vi "Streaming Xcvr (FPGA MODIFIED).vi"() -> ()   [LabVIEW 2015]
doc: "Acquires data from the Rx ports and streams the data to the host while receiving data from the host and generating the resulting waveform at the Tx ports of the NI USRP-294x/295x device. Use this VI as a template for the Simple NI-USRP Streaming sample project."
uses:
  <instrlib>/_niInstr/DSP/v1/Shared/Public/IQ Impairments.ctl
  SubVIs/Stream Control State.ctl
  Host/SubVIs/Start Trigger.ctl
  <instrlib>/_niInstr/DSP/v1/Shared/Public/IQ Gain.ctl
  <instrlib>/_niInstr/Register Bus/v1/FPGA/Public/Read Cmd Data.ctl
  SubVIs/DDC Parameters.ctl
  SubVIs/DUC Parameters.ctl
  <vilib>/Platform/TimedLoop/XDataNode/timing_clust.ctl
  <vilib>/Platform/TimedLoop/XDataNode/nitl_modes.ctl
  <vilib>/Platform/TimedLoop/XDataNode/wakeup.ctl
  <vilib>/rvi/Emulation/niFpgaGetClockAttributes.vi
  <vilib>/rvi/Emulation/niFpgaSctlEmulationGetInTimedLoop.vi
  <vilib>/rvi/Emulation/niFpgaEmulationReportErrorSimple.vi
  <vilib>/rvi/Emulation/niFpgaCriticalErrorInLSC.vi
  <vilib>/rvi/Emulation/niFpgaProcessEmulError.vi
  <vilib>/rvi/eio/common/nirviEmuTemplateMethod_errors.vi
  <vilib>/Platform/TimedLoop/XDataNode/XDataNode.xnode
  <vilib>/eio/EIONode/EIONode.xnode
  <vilib>/Platform/TimedLoop/XDataNode/XDNodeRunTimeDep.lvlib
  <instrlib>/_niInstr/Register Bus/v1/FPGA/niInstr Register Bus v1 FPGA.lvlib
  <instrlib>/_niInstr/DSP/v1/Shared/niInstr DSP v1 Shared.lvlib
  <instrlib>/niUsrpRio/Config/v1/FPGA/niUsrpRio Config v1 FPGA.lvlib
  FPGA Timekeeper.lvlib
  Host/PPS_Global_Var.vi
panel:
  out "FPGA Timekeeper time (ns)":u64
  out "FPGA Timekeeper locked":bool
  out "offset from time reference":i32
  out "PPS":bool
  in  "absolute time offset(ns)":u64
  in  "RF 1/Tx/Enable":bool
  in  "RF 1/Rx/Enable":bool
  in  "RF 0/Tx/Enable":bool
  in  "RF 0/Rx/Enable":bool
  out "tx.parameters":T5={"tx.trigger select"=enum."Software", "tx.trigger enable"=FALSE, "tx.trigger sync enable"=FALSE, "tx 0.stream enable"=FALSE, "tx 1.stream enable"=FALSE, "tx.software trigger"=FALSE, "tx.reset"=FALSE, "tx.abort"=FALSE, "tx.samples to generate"=0, "duc parameters"=[{"frequency shift"=0.0, "impairments"={"inline gain I"=0.0, "inline gain Q"=0.0, "cross gain I"=0.0, "cross gain Q"=0.0, "pre-gain offset I"=0.0, "pre-gain offset Q"=0.0, "post-gain offset I"=0.0, "post-gain offset Q"=0.0}, "phase"=0.0, "input sample rate"=0.0, "gain"={"gain I"=0.0, "gain Q"=0.0}, "delay"=0.0}, {"frequency shift"=0.0, "impairments"={"inline gain I"=0.0, "inline gain Q"=0.0, "cross gain I"=0.0, "cross gain Q"=0.0, "pre-gain offset I"=0.0, "pre-gain offset Q"=0.0, "post-gain offset I"=0.0, "post-gain offset Q"=0.0}, "phase"=0.0, "input sample rate"=0.0, "gain"={"gain I"=0.0, "gain Q"=0.0}, "delay"=0.0}]} {"duc parameters"."frequency shift" format="%#.48g"}
  out "tx.status":T7
  out "rx.status":T8
  out "rx.parameters":T10={"rx.trigger select"=enum."Software", "rx.trigger enable"=FALSE, "rx.trigger sync enable"=FALSE, "rx 0.stream enable"=FALSE, "rx 1.stream enable"=FALSE, "rx.software trigger"=FALSE, "rx.reset"=FALSE, "rx.abort"=FALSE, "rx.samples to acquire"=0, "ddc parameters"=[{"output sample rate"=0.0, "delay"=0.0, "frequency shift"=0.0, "impairments"={"inline gain I"=0.0, "inline gain Q"=0.0, "cross gain I"=0.0, "cross gain Q"=0.0, "pre-gain offset I"=0.0, "pre-gain offset Q"=0.0, "post-gain offset I"=0.0, "post-gain offset Q"=0.0}, "phase"=0.0}, {"output sample rate"=0.0, "delay"=0.0, "frequency shift"=0.0, "impairments"={"inline gain I"=0.0, "inline gain Q"=0.0, "cross gain I"=0.0, "cross gain Q"=0.0, "pre-gain offset I"=0.0, "pre-gain offset Q"=0.0, "post-gain offset I"=0.0, "post-gain offset Q"=0.0}, "phase"=0.0}]} {"ddc parameters"."frequency shift" format="%#.48g"}
  in  "TX DSP Settings Tab Control":T11(tab)=enum."TX Stream Settings"
  in  "tx.trigger enable":bool
  in  "tx.software trigger":bool
  in  "tx.trigger select":T1=enum."Immediate"
  in  "tx.trigger sync enable":bool
  in  "tx 0.stream enable":bool
  in  "tx 1.stream enable":bool
  in  "tx.reset":bool=TRUE
  in  "tx.abort":bool
  in  "tx.samples to generate":u32
  in  "tx.input sample rate":fxp<+,48,1>
  in  "tx.delay":fxp<+/-,18,0>
  out "tx.dsp reset done":bool
  out "tx.state":T6
  out "tx.number of fifo underflows":u32
  out "tx.samples processed":u32
  in  "tx 0.impairments":T3={"inline gain I"=0.9999923706054688, "inline gain Q"=0.9999923706054688, "cross gain I"=0.0, "cross gain Q"=0.0, "pre-gain offset I"=0.0, "pre-gain offset Q"=0.0, "post-gain offset I"=0.0, "post-gain offset Q"=0.0}
  in  "tx 0.frequency shift":fxp<+/-,48,0> format="%#.48g"
  in  "tx 0.phase":fxp<+/-,21,0>
  in  "tx 0.gain":T4={"gain I"=1.0, "gain Q"=1.0}
  out "tx 0.number of IQ data overflows":u64
  in  "tx 1.gain":T4={"gain I"=1.0, "gain Q"=1.0}
  in  "tx 1.phase":fxp<+/-,21,0>
  in  "tx 1.frequency shift":fxp<+/-,48,0> format="%#.48g"
  in  "tx 1.impairments":T3={"inline gain I"=0.9999923706054688, "inline gain Q"=0.9999923706054688, "cross gain I"=0.0, "cross gain Q"=0.0, "pre-gain offset I"=0.0, "pre-gain offset Q"=0.0, "post-gain offset I"=0.0, "post-gain offset Q"=0.0}
  out "tx 1.number of IQ data overflows":u64
  in  "RX DSP Settings Tab Control":T12(tab)=enum."RX Stream Settings "
  in  "rx.trigger enable":bool
  in  "rx.trigger select":T1=enum."Immediate"
  in  "rx.software trigger":bool
  in  "rx.trigger sync enable":bool
  in  "rx.samples to acquire":u32
  out "rx.dsp reset done":bool
  in  "rx.delay":fxp<+/-,16,0>
  in  "rx.output sample rate":fxp<+,48,1>
  out "rx.number of fifo overflows":u32
  out "rx.state":T6
  out "rx.samples processed":u32
  in  "rx.abort":bool
  in  "rx.reset":bool=TRUE
  in  "rx 1.stream enable":bool
  in  "rx 0.stream enable":bool
  in  "rx 0.phase":fxp<+/-,21,0>
  in  "rx 0.frequency shift":fxp<+/-,48,0> format="%#.48g"
  in  "rx 0.impairments":T3={"inline gain I"=0.9999923706054688, "inline gain Q"=0.9999923706054688, "cross gain I"=0.0, "cross gain Q"=0.0, "pre-gain offset I"=0.0, "pre-gain offset Q"=0.0, "post-gain offset I"=0.0, "post-gain offset Q"=0.0}
  out "rx 0.number of IQ data overflows":u64
  in  "rx 1.impairments":T3={"inline gain I"=0.9999923706054688, "inline gain Q"=0.9999923706054688, "cross gain I"=0.0, "cross gain Q"=0.0, "pre-gain offset I"=0.0, "pre-gain offset Q"=0.0, "post-gain offset I"=0.0, "post-gain offset Q"=0.0}
  in  "rx 1.frequency shift":fxp<+/-,48,0> format="%#.48g"
  in  "rx 1.phase":fxp<+/-,21,0>
  out "rx 1.number of IQ data overflows":u64
  in  "reg.host read.go rcvd 0":bool
  out "reg.notify host.go 0":bool
  in  "reg.notify host.go rcvd 0":bool
  out "reg.host read.data 0":T13
  in  "reg.reset 0":bool
  # "FPGA utilization for 120 MS/s"
  # "FPGA utilization for 200 MS/s"
  # "USRP RIO Simple Streaming FPGA"
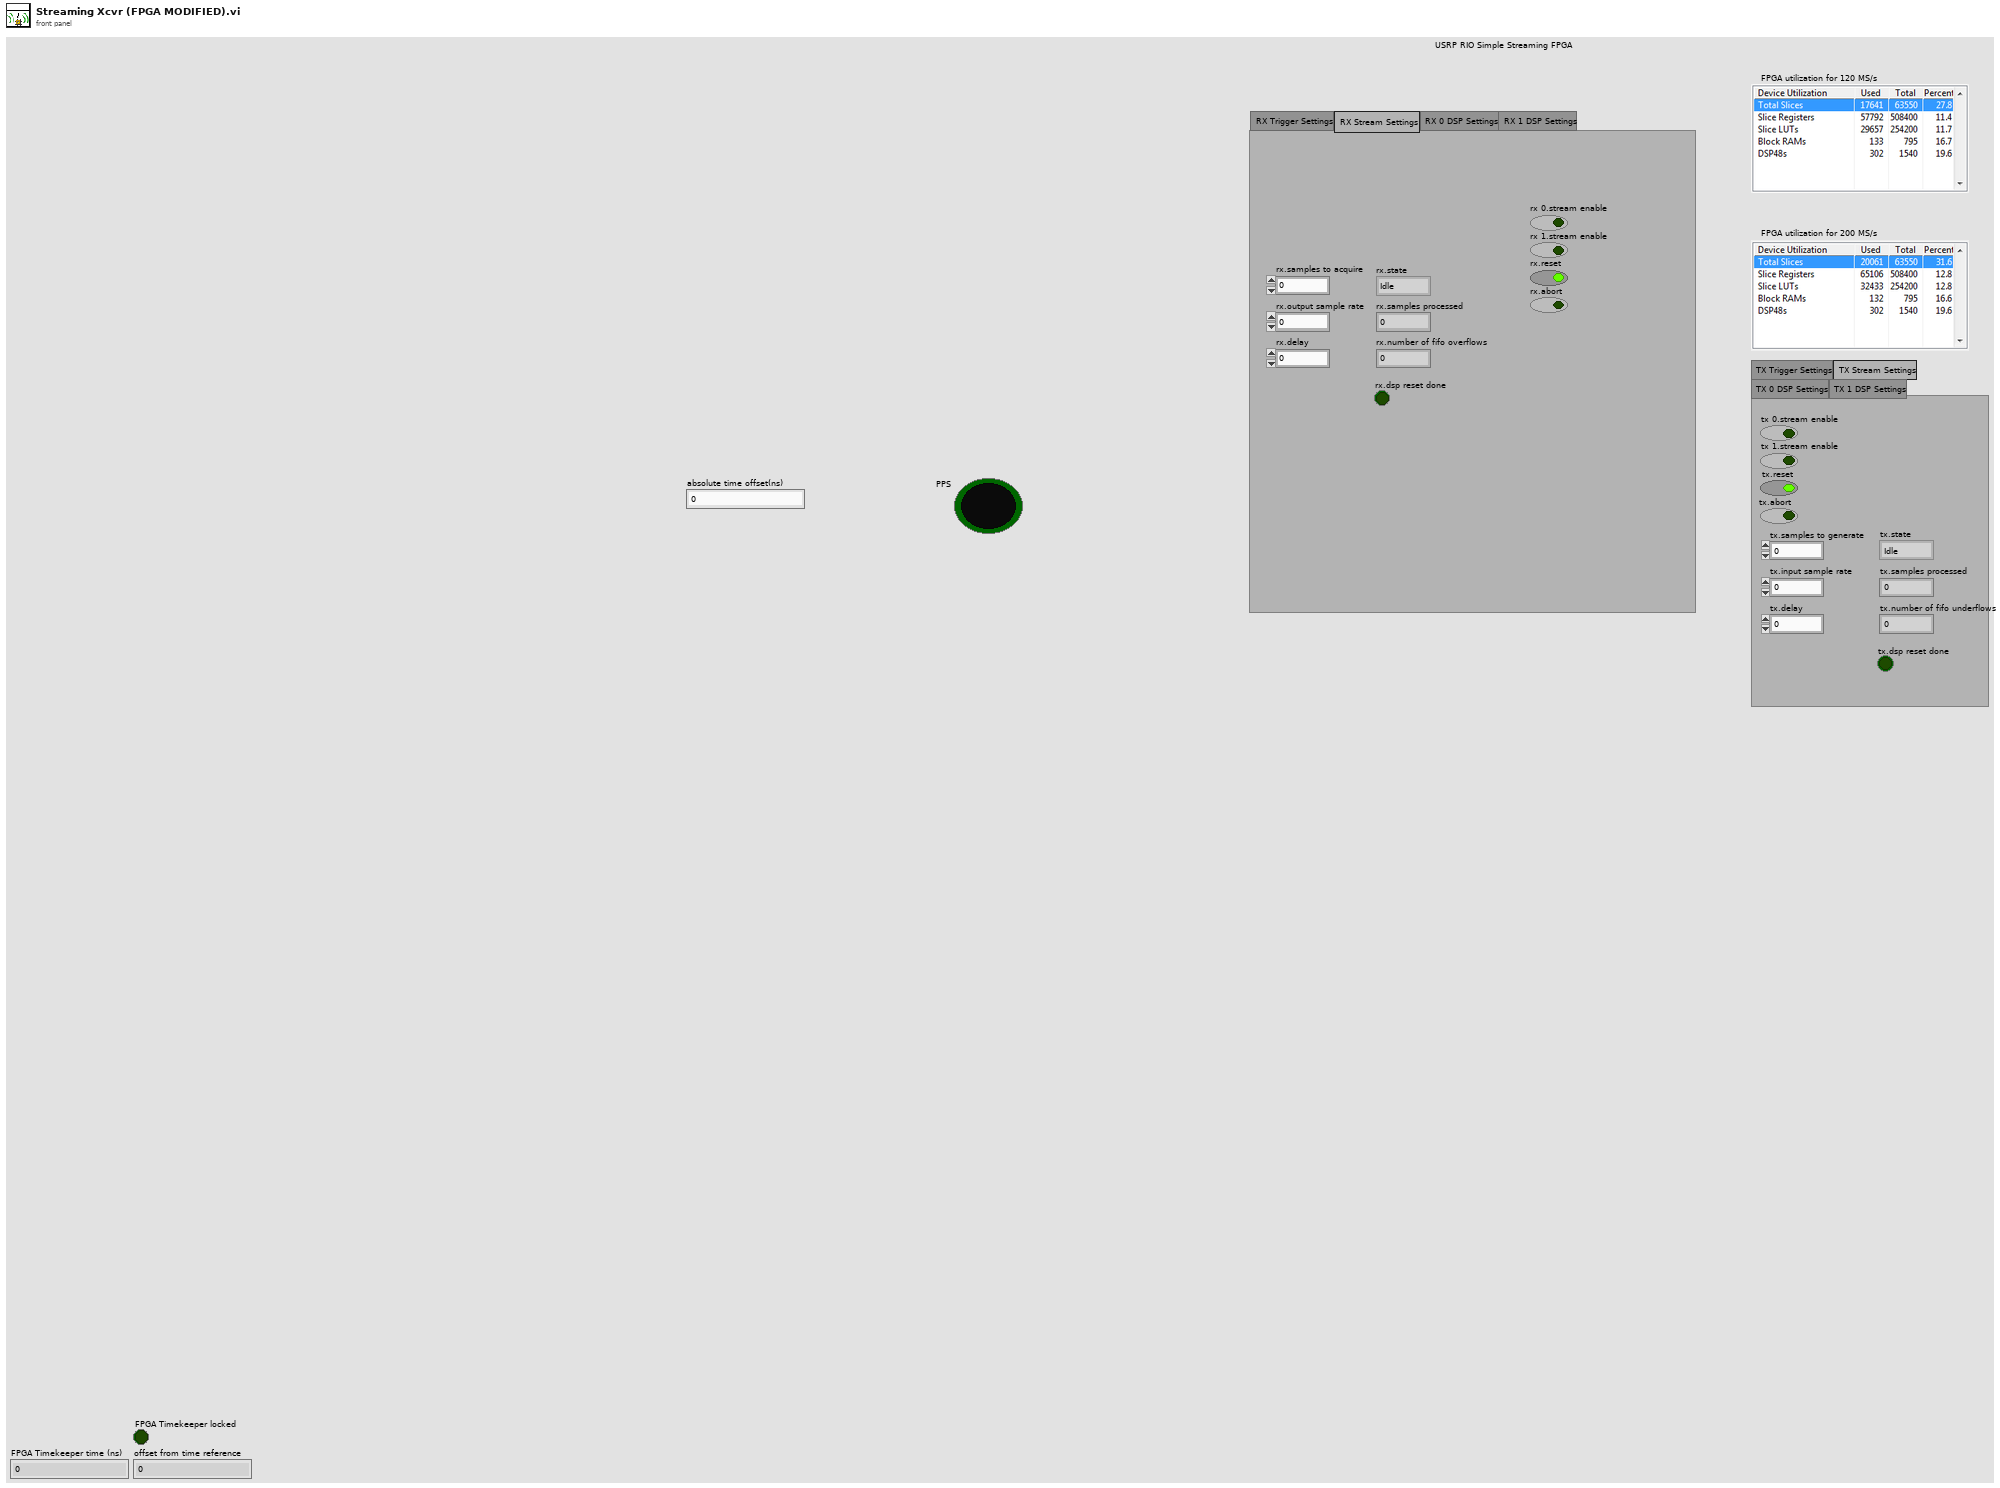
[diagram p1: front panel]
types:
  T1 = typedef "Start Trigger.ctl" = enum8{"Software", "Digital Edge", "Rx Start Trigger", "Tx Start Trigger", "Immediate", "Future Time Event"}
  T2 = typedef "DUC Parameters.ctl" = cluster{"frequency shift":fxp<+/-,48,0>, "impairments":T3, "phase":fxp<+/-,21,0>, "input sample rate":fxp<+,48,1>, "gain":T4, "delay":fxp<+/-,18,0>}
  T3 = typedef "niInstr DSP v1 Shared.lvlib/IQ Impairments.ctl" = cluster{"inline gain I":fxp<+/-,18,1>, "inline gain Q":fxp<+/-,18,1>, "cross gain I":fxp<+/-,18,1>, "cross gain Q":fxp<+/-,18,1>, "pre-gain offset I":fxp<+/-,18,1>, "pre-gain offset Q":fxp<+/-,18,1>, "post-gain offset I":fxp<+/-,18,1>, "post-gain offset Q":fxp<+/-,18,1>}
  T4 = typedef "niInstr DSP v1 Shared.lvlib/IQ Gain.ctl" = cluster{"gain I":fxp<+/-,24,3>, "gain Q":fxp<+/-,24,3>}
  T5 = cluster{"tx.trigger select":T1, "tx.trigger enable":bool, "tx.trigger sync enable":bool, "tx 0.stream enable":bool, "tx 1.stream enable":bool, "tx.software trigger":bool, "tx.reset":bool, "tx.abort":bool, "tx.samples to generate":u32, "duc parameters":T2[]}
  T6 = typedef "Stream Control State.ctl" = enum16{"Idle", "Active"}
  T7 = cluster{"state":T6, "samples processed":u32, "number of fifo underflows":u32, "number of IQ data overflows 0":u64, "number of IQ data overflows 1":u64, "dsp reset done":bool}
  T8 = cluster{"state":T6, "samples processed":u32, "number of fifo overflows":u32, "number of IQ data overflows 0":u64, "number of IQ data overflows 1":u64, "dsp reset done":bool}
  T9 = typedef "DDC Parameters.ctl" = cluster{"output sample rate":fxp<+,48,1>, "delay":fxp<+/-,16,0>, "frequency shift":fxp<+/-,48,0>, "impairments":T3, "phase":fxp<+/-,21,0>}
  T10 = cluster{"rx.trigger select":T1, "rx.trigger enable":bool, "rx.trigger sync enable":bool, "rx 0.stream enable":bool, "rx 1.stream enable":bool, "rx.software trigger":bool, "rx.reset":bool, "rx.abort":bool, "rx.samples to acquire":u32, "ddc parameters":T9[]}
  T11 = enum32{"TX Trigger Settings", "TX Stream Settings", "TX 0 DSP Settings", "TX 1 DSP Settings"}
  T12 = enum32{"RX Trigger Settings", "RX Stream Settings ", "RX 0 DSP Settings", "RX 1 DSP Settings"}
  T13 = typedef "niInstr Register Bus v1 FPGA.lvlib/Read Cmd Data.ctl" = cluster{"go":bool, "data":u32}
  T14 = typedef "XDNodeRunTimeDep.lvlib/timing_clust.ctl" = cluster{"Expected End [f-1]":u64, "Actual End [f-1]":u64, "Finished Late? [f-1]":bool, "Expected End [i-1]":u64, "Actual End [i-1]":u64, "Finished Late? [i-1]":bool, "Expected Start [i]":u64, "Actual Start [i]":u64, "Expected Start [f]":u64, "Actual Start [f]":u64, "Source Name":string, "Structure Name":string, "Period":i64, "Deadline":i64, "Offset":i64, "Start":i64, "Priority":i32, "Timeout":i32, "Mode":T15, "Wakeup Reason":T16, "Error":errorcluster, "Source Type":string, "Secondary Source Type":string, "Global End Time":u64, "Global Start Time":u64, "Frame Duration":u64, "Iteration Duration":u64, "Assigned CPU":i32, "I/O Scan Engine Mode":u32}
  T15 = typedef "XDNodeRunTimeDep.lvlib/nitl_modes.ctl" = enum32{"No Change", "Process missed periods, maintain original phase", "Discard missed periods, maintain original phase", "Process missed periods, ignore original phase", "Discard missed periods, ignore original phase"}
  T16 = typedef "XDNodeRunTimeDep.lvlib/wakeup.ctl" = enum32{"Normal", "Aborted", "Asynchronous wakeup", "Timing source error", "Timed loop error", "Timeout"}
  T17 = cluster{"rx.trigger select":T1, "rx.trigger enable":bool, "rx.trigger sync enable":bool, "rx 0.stream enable":bool, "rx 1.stream enable":bool, "rx.software trigger":bool, "rx.reset":bool, "rx.abort":bool, "rx.samples to acquire":u32, T9[]}
  T18 = cluster{"tx.trigger select":T1, "tx.trigger enable":bool, "tx.trigger sync enable":bool, "tx 0.stream enable":bool, "tx 1.stream enable":bool, "tx.software trigger":bool, "tx.reset":bool, "tx.abort":bool, "tx.samples to generate":u32, T2[]}
  T19 = cluster{"DAC FIFO Reset":refnum<k21>, "RF 0 Rx Swap IQ":refnum<k21>, "RF 0 Rx Negate I":refnum<k21>, "RF 0 Rx Negate Q":refnum<k21>, "RF 0 Rx Data Valid":refnum<k21>, "RF 0 Rx Data Ever Invalid":refnum<k21>, "clear RF 0 Rx Data Ever Invalid":refnum<k21>, "RF 0 Tx Swap IQ":refnum<k21>, "RF 0 Tx Negate I":refnum<k21>, "RF 0 Tx Negate Q":refnum<k21>, "RF 1 Rx Swap IQ":refnum<k21>, "RF 1 Rx Negate I":refnum<k21>, "RF 1 Rx Negate Q":refnum<k21>, "RF 1 Rx Data Valid":refnum<k21>, "RF 1 Rx Data Ever Invalid":refnum<k21>, "clear RF 1 Rx Data Ever Invalid":refnum<k21>, "RF 1 Tx Swap IQ":refnum<k21>, "RF 1 Tx Negate I":refnum<k21>, "RF 1 Tx Negate Q":refnum<k21>}
  T20 = typedef "niUsrpRio Synchronization v1 FPGA.lvlib/Resources.ctl" = cluster{"master":refnum<k21>, "meas.enable":refnum<k21>, "meas.ready":refnum<k21>, "meas.reset":refnum<k21>, "meas.arm":refnum<k21>, "meas.valid":refnum<k21>, "meas.value":refnum<k21>, "meas.oversample factor":refnum<k21>, "cptr":refnum<k21>, "cptr.adjust":refnum<k21>, "cptr.period":refnum<k21>}
  T21 = typedef "niUsrpRio Time v1 FPGA.lvlib/Time Resources.ctl" = cluster{"reset":refnum<k21>, "time":refnum<k21>, "time.previous cptr":refnum<k21>, "new time":refnum<k21>, "new time.when":refnum<k21>, "new time.set":refnum<k21>, "which edge of ref":refnum<k21>, "pps source":refnum<k21>, "internal pps period":refnum<k21>}
  T22 = typedef "niUsrpRio Time v1 FPGA.lvlib/Future Event Resources.ctl" = cluster{"reset":refnum<k21>, "future event.time":refnum<k21>, "future event.ready":refnum<k21>, "future event.set":refnum<k21>, "future event.clear":refnum<k21>, "future event.set in past":refnum<k21>}
  T23 = cluster{"time.resources":T21, "future event.resources":T22, "future event.resources":T22}
  T24 = typedef "niInstr Register Bus v1 FPGA.lvlib/Register Instruction.ctl" = cluster{"subsystem":u8, "address":u16, "data":u32, "valid":bool, "read":bool}
  T25 = typedef "niInstr Register Bus v1 FPGA.lvlib/Read Completion.ctl" = cluster{"data":u32, "valid":bool}
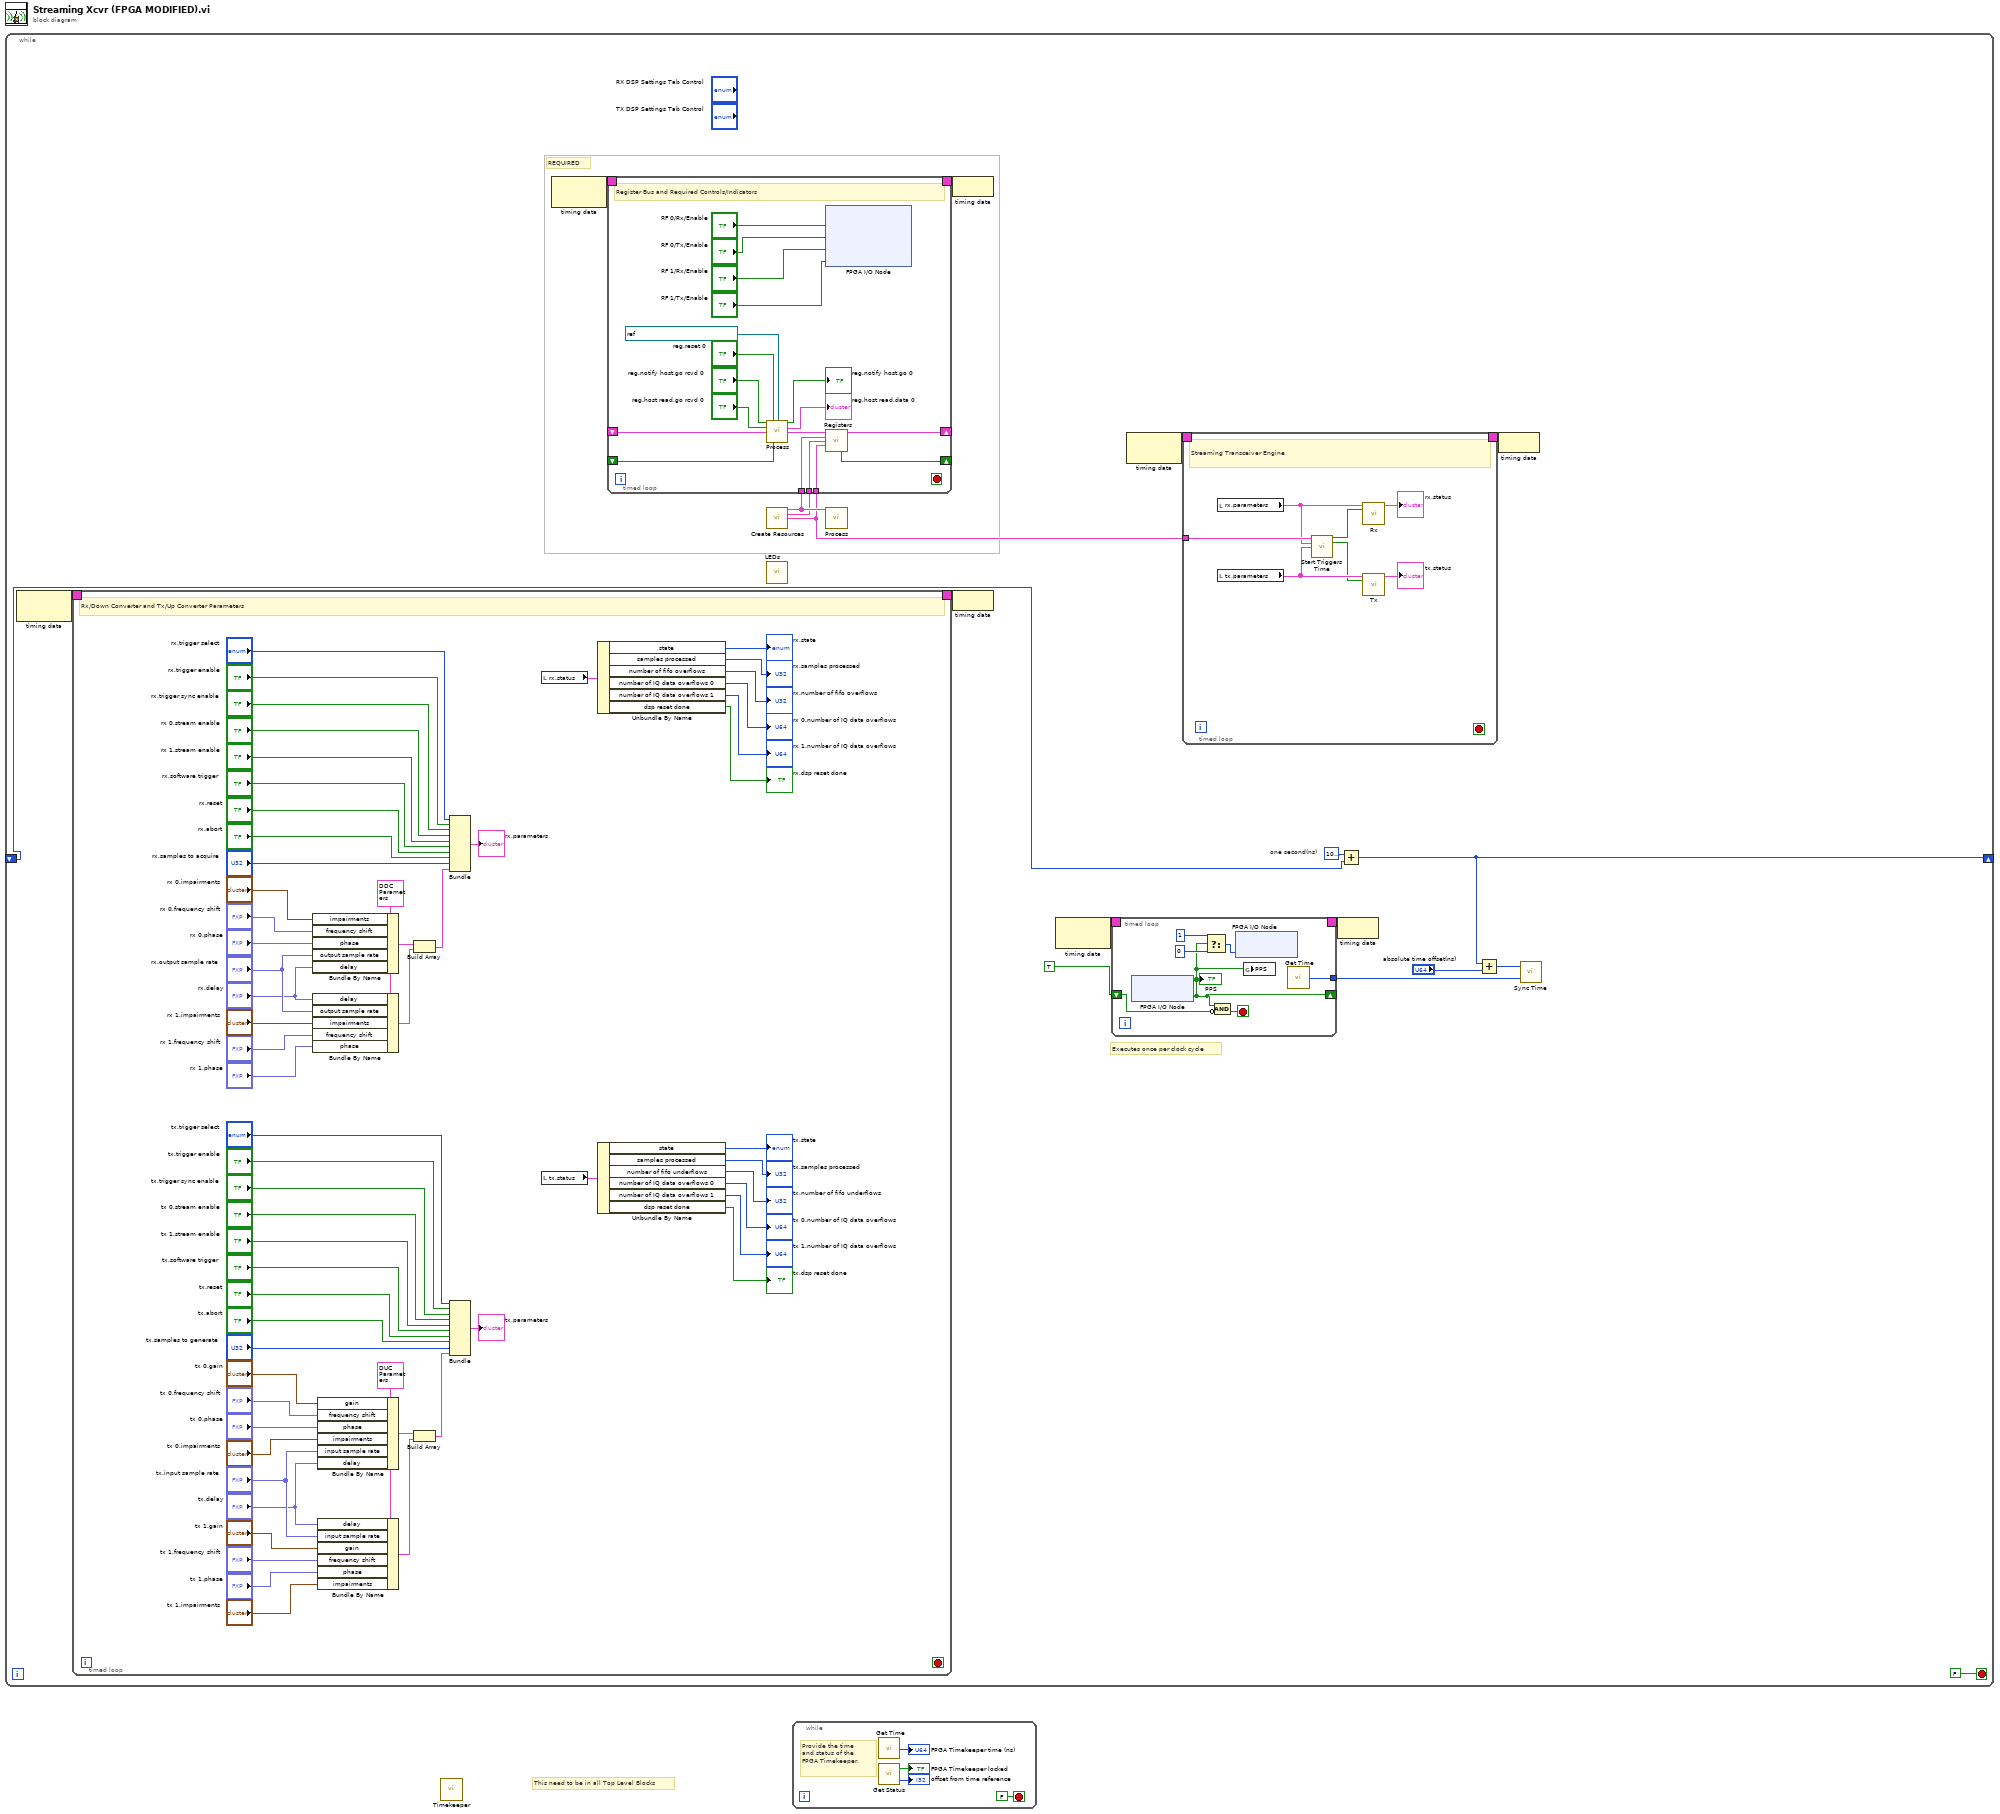
[diagram p0: block diagram]
diagram:
  # "This need to be in all Top Level Blocks"
  n1 = while {
    shift-right: [w2] -> _
    shift-left: _ -> [w1]
    stop <- FALSE stop-if-true
    w3 = u64 1000000000  # one second(ns)
    # "Executes once per clock cycle"
    # "REQUIRED"
    n2 = node-c288() -> (w19:T14)  [unwired: 1 in]
    n3 = timed-loop {
      timing: w19 -> [_]
      timing-out: [_] -> w18
      stop <- _ stop-if-true
      w112 = T2 {"frequency shift"=0.0, "impairments"={"inline gain I"=0.9999923706054688, "inline gain Q"=0.9999923706054688, "cross gain I"=0.0, "cross gain Q"=0.0, "pre-gain offset I"=0.0, "pre-gain offset Q"=0.0, "post-gain offset I"=0.0, "post-gain offset Q"=0.0}, "phase"=0.0, "input sample rate"=0.0, "gain"={"gain I"=1.0, "gain Q"=1.0}, "delay"=0.0} ("DUC Parameters")
      w123 = T9 {"output sample rate"=1.0, "delay"=0.0, "frequency shift"=0.0, "impairments"={"inline gain I"=0.9999923706054688, "inline gain Q"=0.9999923706054688, "cross gain I"=0.0, "cross gain Q"=0.0, "pre-gain offset I"=0.0, "pre-gain offset Q"=0.0, "post-gain offset I"=0.0, "post-gain offset Q"=0.0}, "phase"=0.0} ("DDC Parameters")
      # "Rx/Down Converter and Tx/Up Converter Parameters"
      n4 = Bundle By Name(cluster=w123, "impairments"="rx 0.impairments", "frequency shift"="rx 0.frequency shift", "phase"="rx 0.phase", "output sample rate"="rx.output sample rate", "delay"="rx.delay") -> (w121:T9)
      n5 = Bundle By Name(cluster=w123, "delay"="rx.delay", "output sample rate"="rx.output sample rate", "impairments"="rx 1.impairments", "frequency shift"="rx 1.frequency shift", "phase"="rx 1.phase") -> (w122:T9)
      n6 = Bundle By Name(cluster=w112, "gain"="tx 0.gain", "frequency shift"="tx 0.frequency shift", "phase"="tx 0.phase", "impairments"="tx 0.impairments", "input sample rate"="tx.input sample rate", "delay"="tx.delay") -> (w110:T2)
      n7 = Bundle By Name(cluster=w112, "delay"="tx.delay", "input sample rate"="tx.input sample rate", "gain"="tx 1.gain", "frequency shift"="tx 1.frequency shift", "phase"="tx 1.phase", "impairments"="tx 1.impairments") -> (w111:T2)
      n8 = Build Array(w121, w122) -> (w91:T9[])
      n9 = Build Array(w110, w111) -> (w88:T2[])
      n10 = Bundle("rx.trigger select"="rx.trigger select", "rx.trigger enable"="rx.trigger enable", "rx.trigger sync enable"="rx.trigger sync enable", "rx 0.stream enable"="rx 0.stream enable", "rx 1.stream enable"="rx 1.stream enable", "rx.software trigger"="rx.software trigger", "rx.reset"="rx.reset", "rx.abort"="rx.abort", "rx.samples to acquire"="rx.samples to acquire", w91) -> (→"rx.parameters":T17)  [unwired: 1 in]
      n11 = Bundle("tx.trigger select"="tx.trigger select", "tx.trigger enable"="tx.trigger enable", "tx.trigger sync enable"="tx.trigger sync enable", "tx 0.stream enable"="tx 0.stream enable", "tx 1.stream enable"="tx 1.stream enable", "tx.software trigger"="tx.software trigger", "tx.reset"="tx.reset", "tx.abort"="tx.abort", "tx.samples to generate"="tx.samples to generate", w88) -> (→"tx.parameters":T18)  [unwired: 1 in]
      n12 = local read "rx.status"() -> (w80:T8)
      n13 = local read "tx.status"() -> (w73:T7)
      n14 = Unbundle By Name(w80) -> ("state"=→"rx.state":T6, "samples processed"=→"rx.samples processed":u32, "number of fifo overflows"=→"rx.number of fifo overflows":u32, "number of IQ data overflows 0"=→"rx 0.number of IQ data overflows":u64, "number of IQ data overflows 1"=→"rx 1.number of IQ data overflows":u64, "dsp reset done"=→"rx.dsp reset done":bool)
      n15 = Unbundle By Name(w73) -> ("state"=→"tx.state":T6, "samples processed"=→"tx.samples processed":u32, "number of fifo underflows"=→"tx.number of fifo underflows":u32, "number of IQ data overflows 0"=→"tx 0.number of IQ data overflows":u64, "number of IQ data overflows 1"=→"tx 1.number of IQ data overflows":u64, "dsp reset done"=→"tx.dsp reset done":bool)
    }
    n16 = node-c288() -> (w17:T14)  [unwired: 1 in]
    n17 = call "Create Resources.vi"() -> ("config.resources"=w13:T19, "sync.resources"=w12:T20, "time.resources"=w11:T23)  [unwired: 13 in]
    n18 = timed-loop "Register Bus and Required Controls/Indicators" {
      timing: w17 -> [_]
      timing-out: [_] -> w16
      shift-right: [w56] -> _
      shift-left: _ -> [w55]
      shift-right: [w50] -> _
      shift-left: _ -> [w54]
      tunnel: w13 -> [w48]
      tunnel: w12 -> [w47]
      tunnel: w11 -> [w46]
      stop <- _ stop-if-true
      # "Register Bus and Required Controls/Indicators"
      n19 = call <instrlib>:"Process.vi"("reg.notify host.go rcvd"="reg.notify host.go rcvd 0", "reg.reset"="reg.reset 0", "reg.host instruction fifo"=refnum<k21> "reg.host instruction fifo 0", "reg.host read.go rcvd"="reg.host read.go rcvd 0", "read completion"=w55, "ready for output"=w54) -> ("reg.notify host.go"=→"reg.notify host.go 0":bool, "reg.host read.data"=→"reg.host read.data 0":T13, "register instruction"=w49:T24)  [unwired: 7 in]
      n20 = xnode ("FPGA I/O Node")("RF 0/Rx/Enable"="RF 0/Rx/Enable", "RF 0/Tx/Enable"="RF 0/Tx/Enable", "RF 1/Rx/Enable"="RF 1/Rx/Enable", "RF 1/Tx/Enable"="RF 1/Tx/Enable") -> ()  [unwired: 4 in, 4 out]
      n21 = call "Registers.vi"("register instruction"=w49, "config.resources"=w48, "sync.resources"=w47, "time.resources"=w46) -> ("read completion out"=w56:T25, "ready for input"=w50:bool)  [unwired: 10 in]
    }
    n22 = call "LEDs.vi"() -> ()  [unwired: 1 in]
    n23 = call <instrlib>:"Process.vi"("resources"=w13) -> ()  [unwired: 15 in]
    n24 = node-c288(w16) -> ()
    n25 = node-c288(w18) -> ()
    n26 = node-c288() -> (w9:T14)  [unwired: 1 in]
    n27 = timed-loop {
      timing: w9 -> [_]
      timing-out: [_] -> w8
      shift-right: [w20] -> _
      shift-left: TRUE ("Mod1/DIO0") -> [w26]
      tunnel: [w24] -> w6
      stop <- w25 stop-if-true
      n28 = xnode "FPGA I/O Node"() -> ("GPS PPS"=w20:bool)  [unwired: 1 in, 1 out]
      "PPS" <- w20
      n29 = Select(t=i16 1, s=w20, f=i16 0) -> (s? t:f=w23:i16)
      n30 = Compound Arithmetic op=AND(w20, invert w26) -> (w25:bool)
      n31 = xnode "FPGA I/O Node"("LED/PPS"=w23) -> ()  [unwired: 1 in, 1 out]
      n32 = global write "PPS_Global_Var.vi" "PPS"(w20) -> ()
      n33 = call "Get Time.vi"() -> ("time (ns)"=w24:u64)
    }
    n34 = node-c288() -> (w15:T14)  [unwired: 1 in]
    n35 = timed-loop "Streaming Transceiver Engine" {
      timing: w15 -> [_]
      timing-out: [_] -> w14
      tunnel: w11 -> [w34]
      stop <- _ stop-if-true
      # "Streaming Transceiver Engine"
      n36 = local read "rx.parameters"() -> (w32:T10)
      n37 = local read "tx.parameters"() -> (w33:T5)
      n38 = call "Start Triggers Time.vi"("time.resources"=w34, "rx.parameters"=w32, "tx.parameters"=w33) -> ("rx.start trigger"=w36:bool, "tx.start trigger"=w31:bool)  [unwired: 11 in]
      n39 = call "Rx.vi"("rx.parameters"=w32, "rx.start trigger"=w36) -> ("rx.status"=→"rx.status":T8)  [unwired: 13 in]
      n40 = call "Tx.vi"("tx.parameters"=w33, "tx.start trigger"=w31) -> ("tx.status"=→"tx.status":T7)  [unwired: 13 in]
    }
    n41 = node-c288(w8) -> ()
    n42 = Add(x=w3, y=w1) -> (x+y=w2:u64)
    n43 = Add(x=w2, y="absolute time offset(ns)") -> (x+y=w4:u64)
    n44 = node-c288(w14) -> ()
    n45 = call "Sync Time.vi"("FPGA Timekeeper time (ns)"=w6, "time reference time (ns)"=w4) -> ()
  }
  n46 = call "Timekeeper.vi"() -> ()  [unwired: 12 in]
  n47 = while {
    stop <- FALSE stop-if-true
    # "Provide the time\nand status of the\nFPGA Timekeeper."
    n48 = call "Get Time.vi"() -> ("time (ns)"=→"FPGA Timekeeper time (ns)":u64)
    n49 = call "Get Status.vi"() -> ("FPGA Timekeeper locked"=→"FPGA Timekeeper locked":bool, "offset from time reference"=→"offset from time reference":i32)
  }
